vi "Build_Log_Array.vi"(1 "# Steps":i32, 2 "Max Frequency":u64, 3 "Min Frequency":i64) -> (0 "Array":dbl[](array[numeric]))   [LabVIEW 2012]
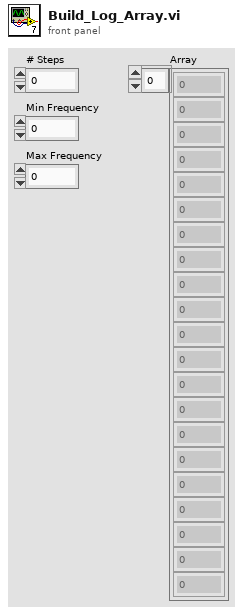
[diagram p1: front panel]
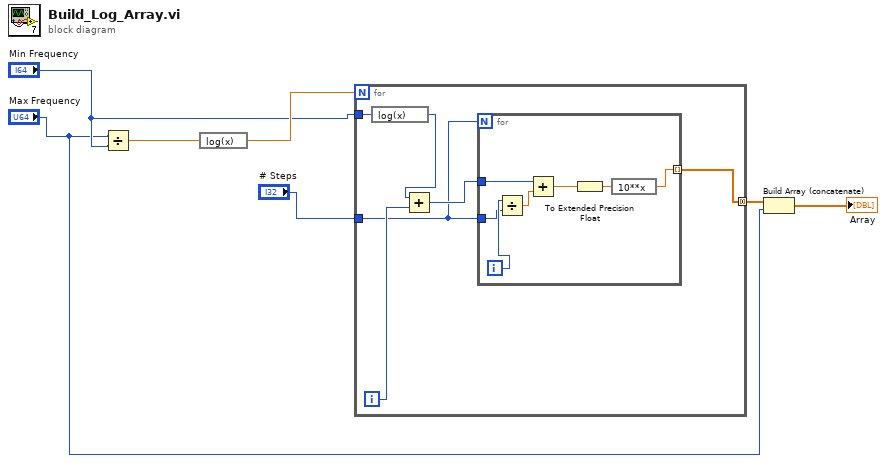
[diagram p0: block diagram]
diagram:
  n1 = Divide(x="Max Frequency", y="Min Frequency") -> (x/y=w7:dbl)
  n2 = expression code="log(x)"(w7) -> (w6:dbl)
  n3 = for {
    N: w6 -> [_]
    tunnel: "Min Frequency" -> [w13]
    tunnel: [w9] -> w4 mode=concatenating
    tunnel: "# Steps" -> [w8]
    i -> [w11]
    n4 = expression code="log(x)"(w13) -> (w12:i64)
    n5 = Add(x=w12, y=w11) -> (x+y=w10:i64)
    n6 = for {
      N: w8 -> [_]
      tunnel: w8 -> [w19]
      tunnel: w10 -> [w17]
      tunnel: [w15] -> w9 mode=indexing
      i -> [w20]
      n7 = Divide(x=w20, y=w19) -> (x/y=w18:dbl)
      n8 = Add(x=w17, y=w18) -> (x+y=w14:dbl)
      n9 = To Extended Precision Float(1:w14) -> (0:w16:ext)
      n10 = expression code="10**x"(w16) -> (w15:ext)
    }
  }
  n11 = Build Array (concatenate)(w4, "Max Frequency") -> (→"Array":ext[])
